vi "Voltage_inputs to x_y_scales.vi"(8 "error in (no error)":errorcluster, 9 "RF meter max.":dbl min=0.0 max=500.0 format="%.2g", 10 "RF meter min.":dbl min=0.0 max=500.0 format="%.2g", 11 "Analog inputs":T1) -> (0 "error out":errorcluster, 2 "y axis value":dbl, 3 "x axis value":dbl)   [LabVIEW 2014]
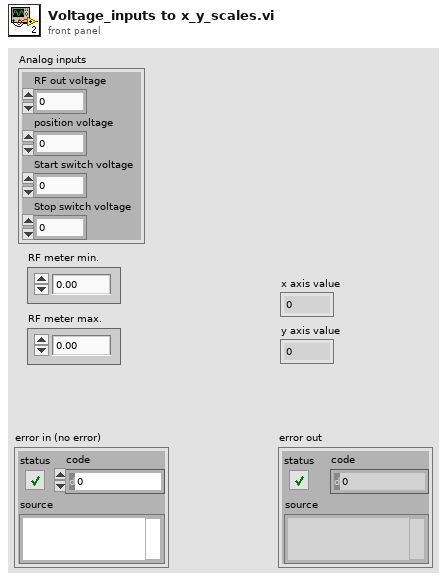
[diagram p1: front panel]
types:
  T1 = cluster{"RF out voltage":dbl, "position voltage":dbl, "Start switch voltage":dbl, "Stop switch voltage":dbl}
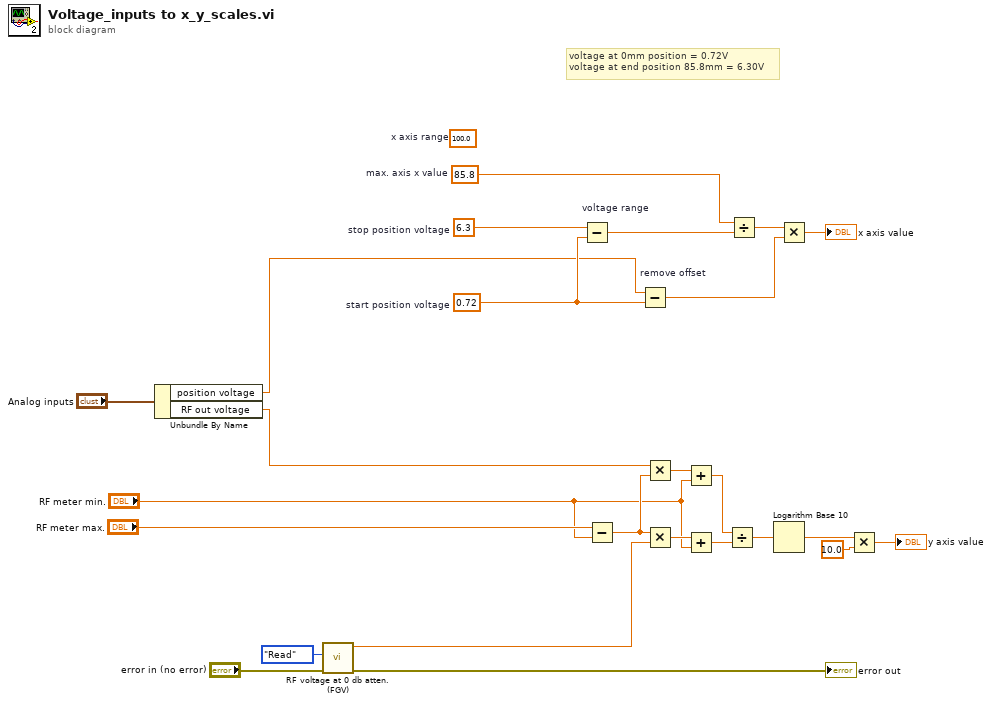
[diagram p0: block diagram]
diagram:
  w1 = 85.8  # max. axis x value
  (unwired) 100.0  # x axis range
  w24 = 0.72  # start position voltage
  w25 = 6.3  # stop position voltage
  # "voltage at 0mm position = 0.72V\nvoltage at end position 85.8mm = 6.30V"
  n1 = Unbundle By Name("Analog inputs") -> ("position voltage"=w15:dbl, "RF out voltage"=w5:dbl)
  n2 = call "RF voltage at 0 db atten. (FGV).vi"("error in (no error)"="error in (no error)", "Enum"=enum16{"Read", "Write"}."Read") -> ("error out"=→"error out":errorcluster, "RF voltage at 0 dB atten."=w2:dbl)  [unwired: 8 in]
  n3 = Subtract "voltage range"(x=w25, y=w24) -> (x-y=w23:dbl)
  n4 = Subtract(x="RF meter max.", y="RF meter min.") -> (x-y=w10:dbl)
  n5 = Subtract "remove offset"(x=w15, y=w24) -> (x-y=w21:dbl)
  n6 = Multiply(x=w5, y=w10) -> (x*y=w12:dbl)
  n7 = Multiply(x=w10, y=w2) -> (x*y=w9:dbl)
  n8 = Add(x=w12, y="RF meter min.") -> (x+y=w11:dbl)
  n9 = Add(x=w9, y="RF meter min.") -> (x+y=w8:dbl)
  n10 = Divide(x=w11, y=w8) -> (x/y=w7:dbl)
  n11 = Divide(x=w1, y=w23) -> (x/y=w22:dbl)
  n12 = Logarithm Base 10(1:w7) -> (0:w14:dbl)
  n13 = Multiply(x=w22, y=w21) -> (x*y=→"x axis value":dbl)
  n14 = Multiply(x=w14, y=10.0) -> (x*y=→"y axis value":dbl)
